vi "Read Limit(Double Float).vi"(7 "Test":string, 8 "error in (no error)":errorcluster) -> (2 "a":dbl, 3 "b":dbl)   [LabVIEW 2019, in "Unit Test Engine Tools.lvlib"]
uses:
  Unit Test Engine Tools.lvlib
  LVUT Global 1.vi
  <vilib>/Utility/file.llb/Read Delimited Spreadsheet (string).vi
panel:
  out "error out":errorcluster
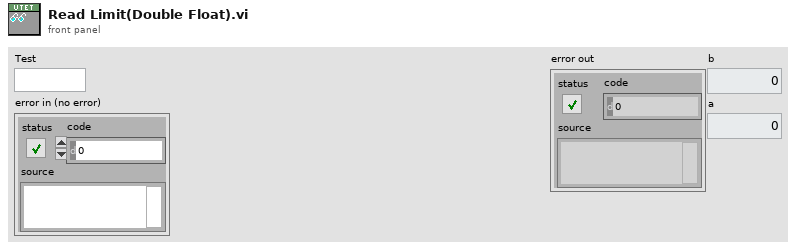
[diagram p1: front panel]
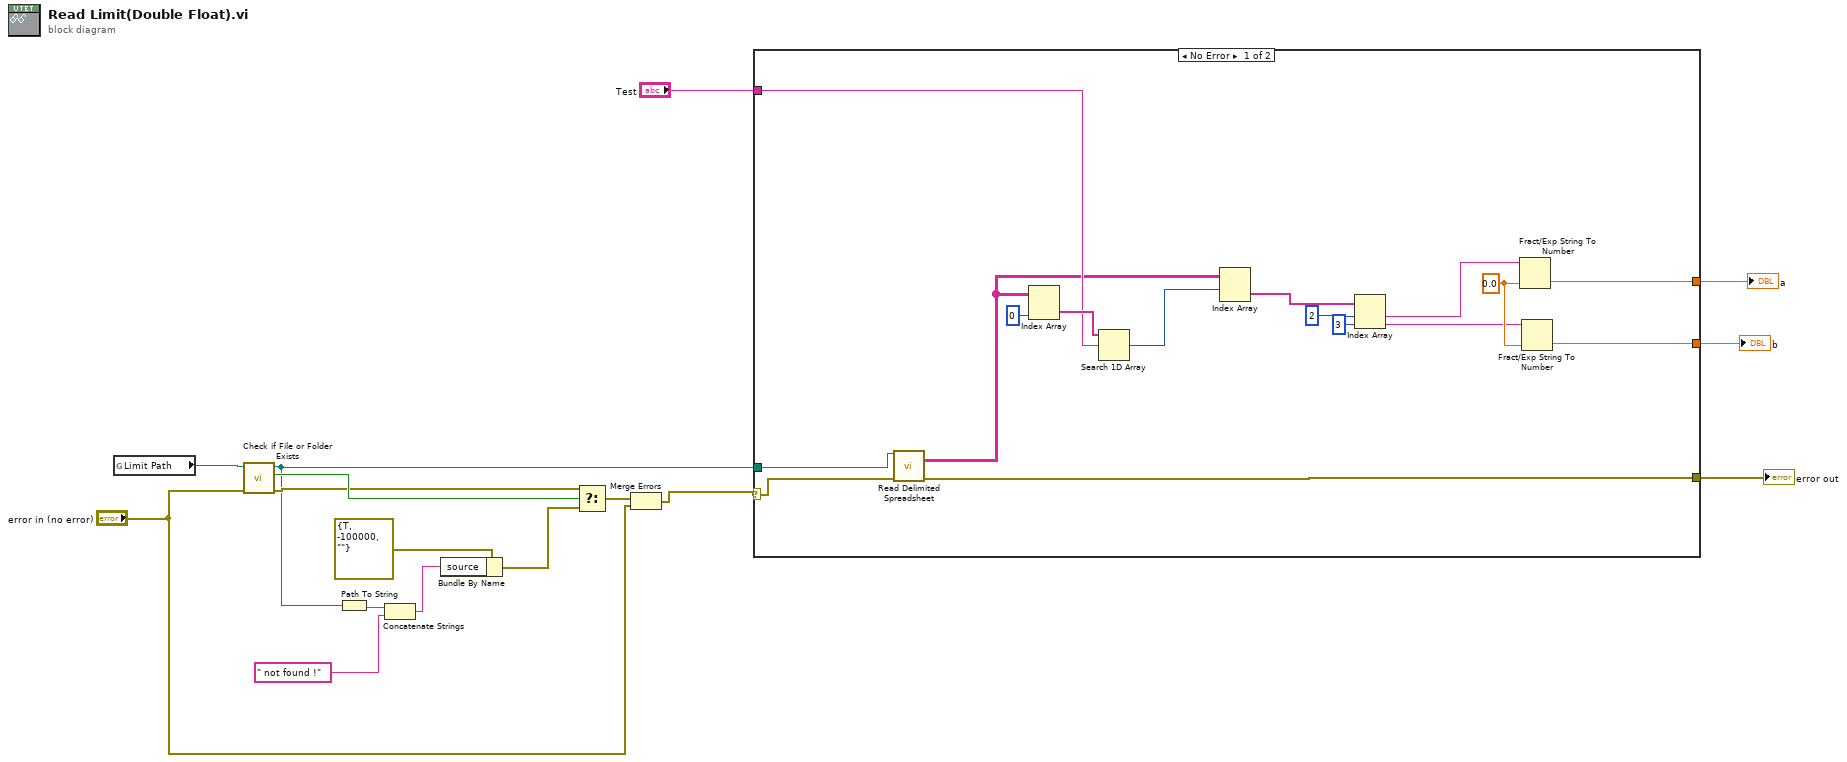
[diagram p0: block diagram]
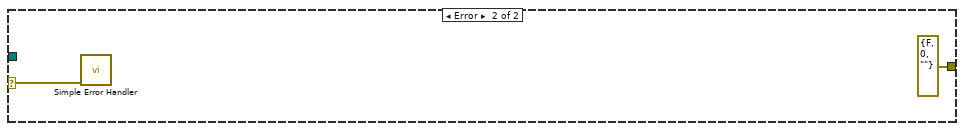
[diagram p2: hidden frame]
diagram:
  n1 = global read "LVUT Global 1.vi" "Limit Path"() -> (w12:path)
  n2 = call <vilib>:"Check if File or Folder Exists.vi"("error in (no error)"="error in (no error)", "path"=w12) -> ("error out"=w10:errorcluster, "file or folder exists?"=w11:bool, "dup path"=w5:path)  [unwired: 7 in]
  n3 = Path To String(path=w5) -> (string=w14:string)
  n4 = Concatenate Strings(w14, " not found !" ("string")) -> (w7:string)
  n5 = Bundle By Name(cluster=errorcluster {"status"=TRUE, "code"=-100000, "source"=""} ("f"), "source"=w7) -> (w8:errorcluster)
  n6 = Select(t=w10, s=w11, f=w8) -> (s? t:f=w6:errorcluster)
  n7 = Merge Errors(w6, "error in (no error)") -> (w4:errorcluster)
  n8 = case shown="No Error" w4 {
    selector: w4 -> [w19 w34]
    tunnel: "Test" -> [w29 _]
    tunnel: [w21 _] -> w1
    tunnel: [w20 _] -> w2
    tunnel: [w18 errorcluster {"status"=FALSE, "code"=0, "source"=""} ("error out")] -> w15
    tunnel: w5 -> [w17 _]
    frame No Error {
      w32 = 0.0 ("default (0 I32)")
      n9 = call-poly <vilib>:"Read Delimited Spreadsheet.vi"("file path (dialog if empty)"=w17, "error in (no error)"=w19) -> ("all rows"=w28:string[][], "error out"=w18:errorcluster)  [unwired: 8 in, 4 out]
      n10 = Index Array(array=w28, index (col)=0 ("disabled index (col)")) -> (element=w30:string[])  [unwired: 1 in]
      n11 = Search 1D Array(1D array=w30, element=w29) -> (index of element=w27:i32)  [unwired: 1 in]
      n12 = Index Array(array=w28, index (row)=w27) -> (element=w26:string[])  [unwired: 1 in]
      n13 = Index Array(array=w26, index #1=2 ("index"), index #2=3 ("index")) -> (element #1=w23:string, element #2=w22:string)
      n14 = Fract/Exp String To Number(string=w23, default (0 dbl)=w32) -> (number=w21:dbl)  [unwired: 2 in, 1 out]
      n15 = Fract/Exp String To Number(string=w22, default (0 dbl)=w32) -> (number=w20:dbl)  [unwired: 2 in, 1 out]
    }
    frame Error {
      n16 = call <vilib>:"Simple Error Handler.vi"("error in (no error)"=w34) -> ()  [unwired: 4 in, 5 out]
    }
  }
  "b" <- w2
  "a" <- w1
  "error out" <- w15
